vi "GlobalClicksHeight.vi"() -> ()   [LabVIEW 2019]
panel:
  in  "Calibrated?":bool
  in  "Starting Height?":bool
  in  "Clicks and Height":bool
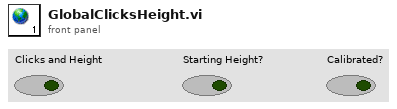
[diagram p1: front panel]
diagram:
